vi "Get Panel from SubPanel.vi"(7 "Panel Type (Panel)":refnum<class "Panel.lvclass">, 8 "error in (no error)":errorcluster, 10 "SubPanel":refnum<vi>, 11 "Manager in":refnum<class "Manager.lvclass">) -> (0 "error out":errorcluster, 1 "Has Panel":bool, 2 "Panel":refnum<class "Panel.lvclass">, 3 "Manager out":refnum<class "Manager.lvclass">)   [LabVIEW 2020, in "OOPanel.lvlib" / "Manager.lvclass"]
uses:
  Manager.lvclass
  Panel/Panel.lvclass
  Manager.lvclass/Manager.ctl
  <vilib>/Utility/error.llb/Error Cluster From Error Code.vi
  <vilib>/ErrorRing/Error Ring.xnode
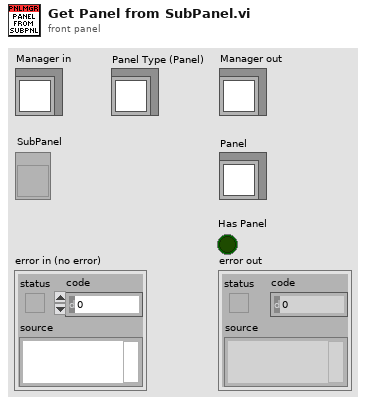
[diagram p1: front panel]
types:
  T1 = typedef "OOPanel.lvlib/Manager.lvclass/Ref Data.ctl" = cluster{"Created Panels":refnum<class "Panel.lvclass">[], "Subpanel Map":map{refnum<vi>, T2}}
  T2 = typedef "OOPanel.lvlib/Manager.lvclass/Subpanel Data.ctl" = cluster{"Panel":refnum<class "Panel.lvclass">, "Has Panel":bool, "Visible":bool}
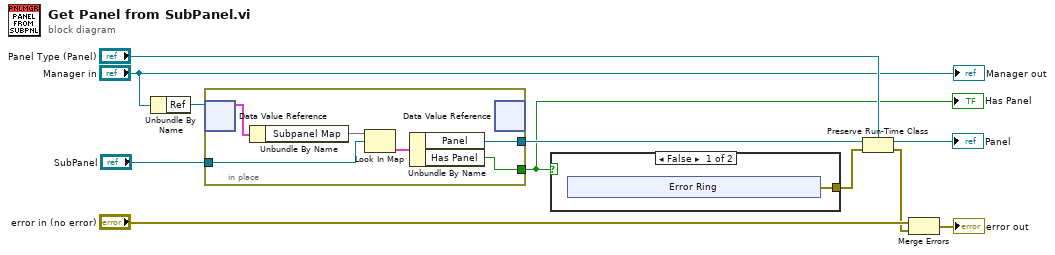
[diagram p0: block diagram]
diagram:
  n1 = Unbundle By Name("Manager in") -> ("Ref"=w10:refnum<data-value>)
  n2 = in-place {
    in-place-border: "SubPanel" -> [w15]
    in-place-border: [w13] -> w8
    in-place-border: [w12] -> w1
    n3 = in-place-dvr #1(w10) -> (w17:T1)  [unwired: 1 out]
    n4 = Unbundle By Name(w17) -> ("Subpanel Map"=w16:map{refnum<vi>, T2})
    n5 = Look In Map(map=w16, key=w15) -> (value=w14:T2)  [unwired: 1 in, 1 out]
    n6 = Unbundle By Name(w14) -> ("Panel"=w13:refnum<class "Panel.lvclass">, "Has Panel"=w12:bool)
    n7 = in-place-dvr #1() -> ()  [unwired: 1 in, 2 out]
  }
  "Has Panel" <- w1
  n8 = case shown="False" w1 {
    tunnel: [w18 _] -> w3
    frame False {
      n9 = xnode "Error Ring"() -> ("error out"=w18:errorcluster)
    }
    frame True {
    }
  }
  n10 = Preserve Run-Time Class(object in=w8, error in=w3, 2:"Panel Type (Panel)") -> (object out=→"Panel":refnum<class "Panel.lvclass">, error out=w4:errorcluster)
  n11 = Merge Errors("error in (no error)", w4) -> (→"error out":errorcluster)
  "Manager out" <- "Manager in"
